vi "Abort Motion.vi"(4 "error in (no error)":errorcluster, 7 "VISA resource name":refnum<visa-resource-name>) -> (0 "error out":errorcluster, 3 "VISA resource name out":refnum<visa-resource-name>)   [LabVIEW 2020, in "Newport ESP301.lvlib"]
doc: "This command should be used as an emergency stop. On reception of this\ncommand, the controller invokes emergency stop event processing for each axis as configured by ZE (e-stop event configuration) command.\nBy default axes are configured to turn motor power OFF, however, individual axes can be configured to stop using emergency deceleration rate set by AE command and maintain motor power.\nIt should be used only as an immediate command, not in a program.\n<B>NOTE:</B> This command affects all axes, however the action taken is determined by each individual’s axis ZE command configuration."
uses:
  Newport ESP301.lvlib
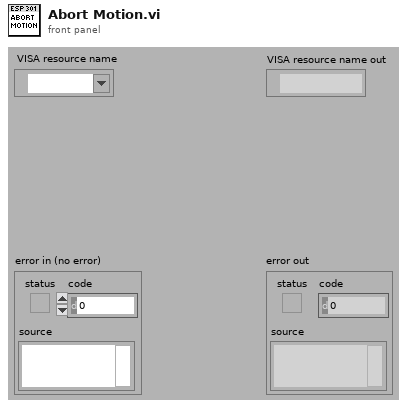
[diagram p1: front panel]
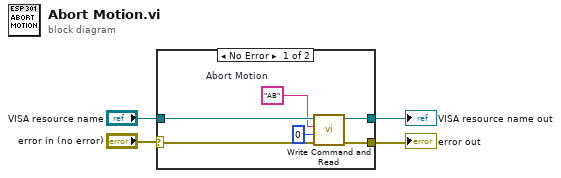
[diagram p0: block diagram]
diagram:
  n1 = case shown="No Error" "error in (no error)" {
    selector: "error in (no error)" -> [w7 w12]
    tunnel: [w9 w12] -> w4
    tunnel: "VISA resource name" -> [w10 w11]
    tunnel: [w8 w11] -> w3
    frame No Error {
      w5 = "AB"  # Abort Motion
      n2 = call "Write Command and Read.vi"("error in (no error)"=w7, "Bytes to read (100)"=u32 0, "Command"=w5, "VISA resource name"=w10) -> ("error out"=w9:errorcluster, "VISA resource name out"=w8:refnum<visa-resource-name>)  [unwired: 1 in, 3 out]
    }
    frame Error {
    }
  }
  "error out" <- w4
  "VISA resource name out" <- w3
